vi "New Data.vi"(6 "dt":dbl, 8 "error in (no error)":errorcluster, 9 "t0":dbl, 10 "Data":dbl[][](array[numeric]), 11 "DataHandlerTask in":refnum<class "DataHandlerTask.lvclass">) -> (0 "error out":errorcluster, 3 "DataHandlerTask out":refnum<class "DataHandlerTask.lvclass">)   [LabVIEW 2020, in "VolatusData.lvlib" / "DataHandlerTask.lvclass"]
uses:
  DataHandlerTask.lvclass
  Volatus/Task/Task.lvclass
  C:/dev/lv20CE/relink/lv-volatus/Volatus/Task/Task.lvclass
  C:/Program Files (x86)/National Instruments/LabVIEW 2020/vi.lib/ActorFramework/Actor/Actor.lvclass
  C:/dev/lv20CE/relink/lv-volatus/Volatus/TaskStateHandler/TaskStateHandler.lvclass
  C:/dev/lv20CE/relink/lv-volatus/Volatus/VectoMessageHandler/VectoMessageHandler.lvclass
  C:/dev/lv20CE/relink/lv-volatus/Volatus/DataHandlerTask/DataHandlerTask.lvclass
  C:/dev/lv20CE/relink/lv-volatus/Volatus/API Provider/API Provider.lvclass
  C:/dev/lv20CE/relink/lv-volatus/Volatus/DataHandler/DataHandler.lvclass
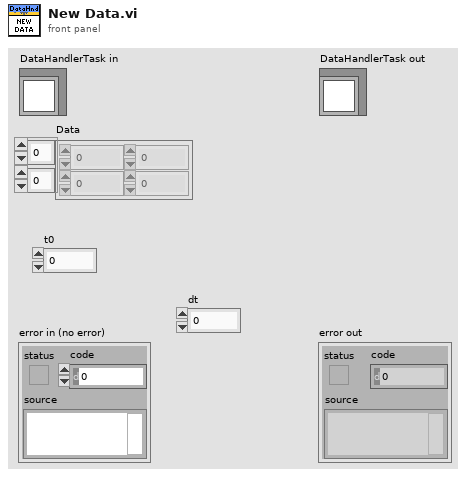
[diagram p1: front panel]
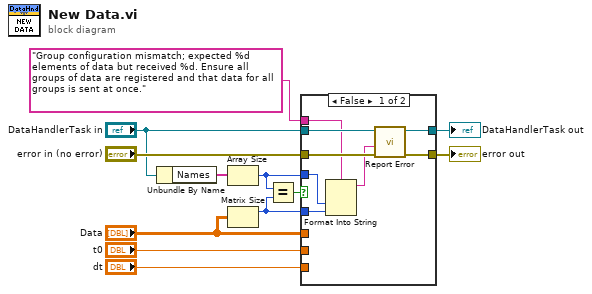
[diagram p0: block diagram]
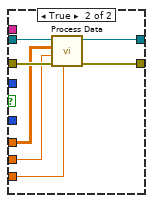
[diagram p2: hidden frame]
diagram:
  n1 = Unbundle By Name("DataHandlerTask in") -> ("Names"=w11:string[])
  n2 = Array Size(array=w11) -> (size(s)=w4:i32)
  n3 = Matrix Size(0:"Data") -> (1:w5:i32)  [unwired: 1 out]
  n4 = Equal?(x=w4, y=w5) -> (x = y?=w7:bool)
  n5 = case shown="False" w7 {
    tunnel: "error in (no error)" -> [w20 w27]
    tunnel: [w19 w26] -> w10
    tunnel: [w17 w23] -> w9
    tunnel: "DataHandlerTask in" -> [w18 w25]
    tunnel: "Data" -> [_ w24]
    tunnel: w5 -> [w14 _]
    tunnel: w4 -> [w15 _]
    tunnel: "t0" -> [_ w22]
    tunnel: "dt" -> [_ w21]
    tunnel: "Group configuration mismatch; expected %d elements of data but received %d. Ensure all groups of data are registered and that data for all groups is sent at once." -> [w13 _]
    frame False {
      n6 = Format Into String(format string=w13, w15, w14) -> (resulting string=w16:string)  [unwired: 2 in, 1 out]
      n7 = call "Report Error.vi"("error in (no error)"=w20, "Message"=w16, "Task in"=w18) -> ("error out"=w19:errorcluster, "Task in"=w17:refnum<class "DataHandlerTask.lvclass">)  [unwired: 7 in]
    }
    frame True {
      n8 = call-dynamic "Process Data.vi"("dt"=w21, "error in (no error)"=w27, "t0"=w22, "Data"=w24, "DataHandlerTask in"=w25) -> ("error out"=w26:errorcluster, "DataHandlerTask out"=w23:refnum<class "DataHandlerTask.lvclass">)  [unwired: 5 in]
    }
  }
  "error out" <- w10
  "DataHandlerTask out" <- w9
